vi "TransformString.vi"(8 "error in (no error)":errorcluster, 10 "String":string, 11 "UnaryOperator in":refnum<class "UnaryOperator.lvclass">) -> (0 "error out":errorcluster, 2 "String out":string, 3 "UnaryOperator out":refnum<class "UnaryOperator.lvclass">)   [LabVIEW 2017, in "Constraint.lvlib" / "UnaryOperator.lvclass"]
doc: "Transforms the string returned by the member constraint's <B>ToString</B> or <B>FailureDescription</B> such that it reflects the operation of this expression."
uses:
  UnaryOperator.lvclass
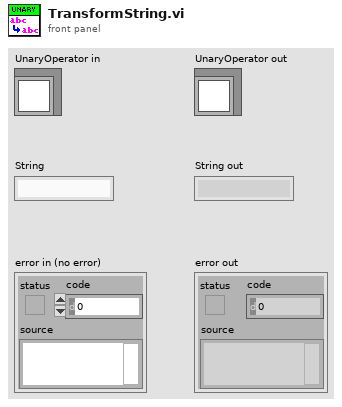
[diagram p1: front panel]
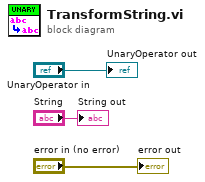
[diagram p0: block diagram]
diagram:
  "error out" <- "error in (no error)"
  "UnaryOperator out" <- "UnaryOperator in"
  "String out" <- "String"
